vi "Set Acquisition Interval.vi"(7 "Client parameters":cluster{"IP":string, "Port":u16}={"IP"="28.0.0.0", "Port"=6666}, 8 "Error In":errorcluster, 10 "Acquisition interval [ms]":i32=50 min=10 max=640 step=10 format="%.0fms", 11 "connection ID":refnum<k16>) -> (0 "Error Out":errorcluster, 3 "connection ID out":refnum<k16>)   [LabVIEW 2016, in "MKR1000.lvlib"]
doc: "This VI sets the Acquisition interval between two points. Lower times causes faster acquisition rate. The VI try 5 times to receive ACKnowledgment for the sent command before returning Error 5000.\n\nNOTE:\nThe MKR1000 VI Library uses UDP. UDP is a connectionless protocol. With the term \"connection\" is intended that MKR1000 gives back an ACKnoledgment packet for each command sent. If no packet is returned (MKR1000 not connected to the net, out of range, etc.), the command is intended LOST and the VIs attempts to send the command again few times before returning Error 5000"
uses:
  MKR1000.lvlib
  Typedef/MKR1000 - Commands.ctl
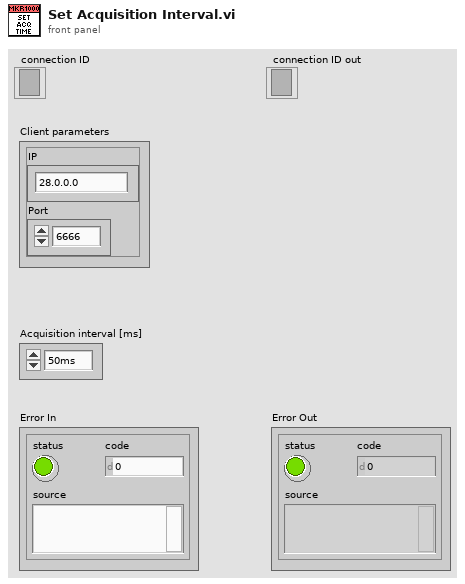
[diagram p1: front panel]
types:
  T1 = typedef "MKR1000.lvlib/MKR1000 - Commands.ctl" = string
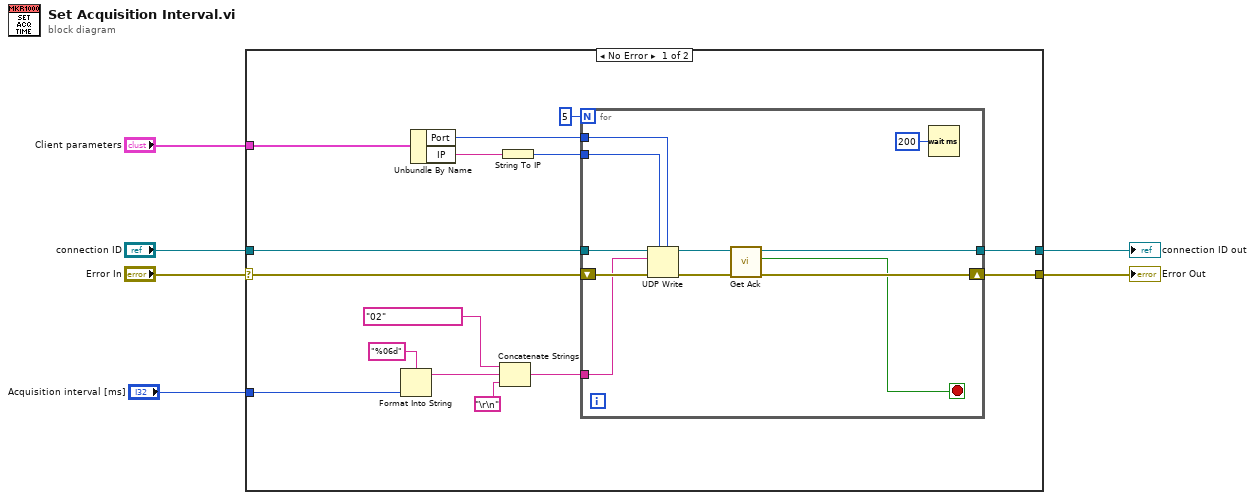
[diagram p0: block diagram]
diagram:
  n1 = case shown="No Error" "Error In" {
    selector: "Error In" -> [w15 w34]
    tunnel: "connection ID" -> [w20 w33]
    tunnel: "Client parameters" -> [w19 _]
    tunnel: [w14 w34] -> w3
    tunnel: [w16 w33] -> w2
    tunnel: "Acquisition interval [ms]" -> [w9 _]
    frame No Error {
      n2 = Format Into String(format string="%06d", w9) -> (resulting string=w10:string)  [unwired: 2 in, 1 out]
      n3 = Unbundle By Name(w19) -> ("Port"=w17:u16, "IP"=w18:string)
      n4 = Concatenate Strings(T1 "02" ("Combo Box"), w10, "\r\n") -> (w8:string)
      n5 = String To IP(1:w18) -> (0:w21:u32)
      n6 = for {
        N: 5 -> [_]
        tunnel: w21 -> [w32]
        tunnel: w17 -> [w30]
        tunnel: w8 -> [w28]
        shift-right: [w24] -> w14
        shift-left: w15 -> [w29]
        tunnel: w20 -> [w31]
        tunnel: [w26] -> w16
        stop <- w23 stop-if-true
        n7 = UDP Write(address=w32, port or service name=w30, connection ID=w31, data in=w28, 8:w29) -> (error out=w25:errorcluster, 3:w27:refnum<k16>)  [unwired: 1 in]
        n8 = call "Get Ack.vi"("Error In"=w25, "connection ID"=w27) -> ("Error Out"=w24:errorcluster, "Ack status"=w23:bool, "connection ID out"=w26:refnum<k16>)  [unwired: 7 in]
        n9 = Wait (ms)(milliseconds to wait=u32 200) -> ()  [unwired: 1 out]
      }
    }
    frame Error {
    }
  }
  "Error Out" <- w3
  "connection ID out" <- w2
